vi "CAN_Close.vi"(8 "error in":errorcluster, 11 "CAN Jaguars Ref":T1) -> (0 "error out":errorcluster)   [LabVIEW 2009, in "OWNCAN.lvlib"]
doc: "Closes the CAN interface."
uses:
  OWNCAN.lvlib
  CAN Jaguars Ref.ctl
  CAN/SubVIs/CAN Jaguar Ref.ctl
  CAN/SubVIs/CAN Jaguar Control Mode.ctl
  CAN.lvlib
  Serial.lvlib
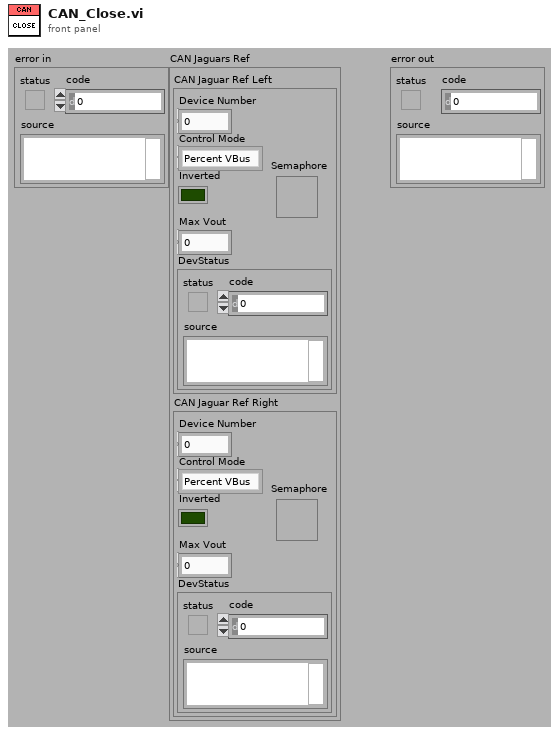
[diagram p1: front panel]
types:
  T1 = typedef "OWNCAN.lvlib/CAN Jaguars Ref.ctl" = cluster{"CAN Jaguar Ref Left":T2, "CAN Jaguar Ref Right":T2}
  T2 = typedef "CAN.lvlib/CAN Jaguar Ref.ctl" = cluster{"Device Number":u8, "Control Mode":T3, "Inverted":bool, "Semaphore":T4, "Max Vout":dbl, "DevStatus":errorcluster}
  T3 = typedef "CAN.lvlib/CAN Jaguar Control Mode.ctl" = enum16{"Percent VBus", "Speed", "Position", "Current"}
  T4 = typedef "Semaphore RefNum" = refnum<k1>
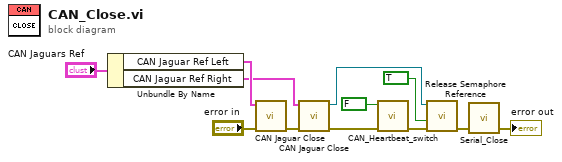
[diagram p0: block diagram]
diagram:
  n1 = Unbundle By Name("CAN Jaguars Ref") -> ("CAN Jaguar Ref Left"=w11:T2, "CAN Jaguar Ref Right"=w10:T2)
  n2 = call "CAN Jaguar Close.vi"("error in (no error)"="error in", "CAN Jaguar Ref"=w11) -> ("error out"=w6:errorcluster)  [unwired: 8 in, 1 out]
  n3 = call "CAN Jaguar Close.vi"("error in (no error)"=w6, "CAN Jaguar Ref"=w10) -> ("error out"=w5:errorcluster, "Semaphore"=w4:T4)  [unwired: 8 in]
  n4 = call "CAN_Heartbeat_switch.vi"("error in"=w5, "Enable? (T)"=FALSE ("CAN_Hearbeat_boolVar")) -> ("error out"=w2:errorcluster)  [unwired: 9 in]
  n5 = call <vilib>:"Release Semaphore Reference.vi"("error in (no error)"=w2, "force destroy? (F)"=TRUE, "semaphore"=w4) -> ("error out"=w1:errorcluster)  [unwired: 7 in, 1 out]
  n6 = call "Serial_Close.vi"("error in (no error)"=w1) -> ("error out"=→"error out":errorcluster)  [unwired: 4 in]
